vi "Read Async Status Queue.vi"(8 "error in (no error)":errorcluster, 10 "timeout in ms (0)":i32, 11 "Async Status in":refnum<queue>) -> (0 "error out":errorcluster, 2 "State":T1, 3 "Async Status out":refnum<queue>)   [LabVIEW 2012, in "Waveform Data Logger Engine.lvlib"]
uses:
  Waveform Data Logger Engine.lvlib
  Types/Async Status.ctl
  Types/Async State.ctl
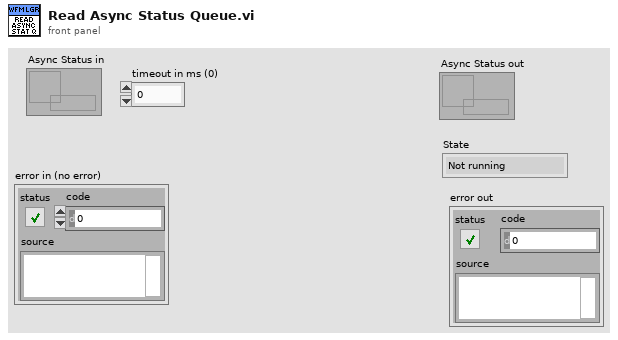
[diagram p1: front panel]
types:
  T1 = typedef "Waveform Data Logger Engine.lvlib/Async State.ctl" = enum16{"Not running", "Initializing", "Running", "Stopped"}
  T2 = typedef "Waveform Data Logger Engine.lvlib/Async Status.ctl" = cluster{"State":T1, "error":errorcluster}
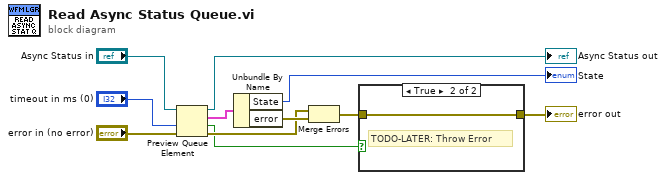
[diagram p0: block diagram]
diagram:
  n1 = Preview Queue Element(queue="Async Status in", timeout in ms (-1)="timeout in ms (0)", error in (no error)="error in (no error)") -> (queue out=→"Async Status out":refnum<queue>, element=w8:T2, timed out?=w3:bool, error out=w5:errorcluster)
  n2 = Unbundle By Name(w8) -> ("State"=→"State":T1, "error"=w6:errorcluster)
  n3 = Merge Errors(w5, w6) -> (w2:errorcluster)
  n4 = case shown="True" w3 {
    tunnel: w2 -> [w12 w13]
    tunnel: [w12 w13] -> w1
    frame False {
    }
    frame True {
      # "TODO-LATER: Throw Error"
    }
  }
  "error out" <- w1
